vi "Stop Acquisition.vi"(8 "error in (no error)":errorcluster, 11 "Cluster":T1={"Camera.lvclass"=refnum, "InClusTiming 2"={"Pixelclock"=24, "Exposure"=46.39115, "ExposureTimeBase"=2, "Framerate"=14.99615, "TriggerMode"=0}, "ROI"={"PosX"=0, "PosY"=0, "Width"=0, "Height"=0}, "File Path Control"=path "", "mirror.lvclass"=refnum} {"InClusTiming 2"."TriggerMode" items=["Auto", "Software", "External sequence start ", "External exposure control"]; "InClusTiming 2"."ExposureTimeBase" items=["nanoseconds", "microseconds", "milliseconds"]; "InClusTiming 2"."Pixelclock" min=1 max=400 step=1 scale=0.05915..400.0 scale format="%#.3g"; "InClusTiming 2"."Framerate" min=0.05915 max=2000.0 step=1.0 scale=0.05915..100.0 scale format="%#.3g"; "InClusTiming 2"."Exposure" min=0.05915 max=2000.0 step=1.0 scale=0.05915..100.0 scale format="%#.3g"}) -> (0 "error out":errorcluster, 3 "Cluster":T1={"Camera.lvclass"=refnum, "InClusTiming 2"={"Pixelclock"=24, "Exposure"=46.39115, "ExposureTimeBase"=2, "Framerate"=14.99615, "TriggerMode"=0}, "ROI"={"PosX"=0, "PosY"=0, "Width"=0, "Height"=0}, "File Path Control"=path "", "mirror.lvclass"=refnum} {"InClusTiming 2"."TriggerMode" items=["Auto", "Software", "External sequence start ", "External exposure control"]; "InClusTiming 2"."ExposureTimeBase" items=["nanoseconds", "microseconds", "milliseconds"]; "InClusTiming 2"."Pixelclock" min=1 max=400 step=1 scale=0.05915..400.0 scale format="%#.3g"; "InClusTiming 2"."Framerate" min=0.05915 max=2000.0 step=1.0 scale=0.05915..100.0 scale format="%#.3g"; "InClusTiming 2"."Exposure" min=0.05915 max=2000.0 step=1.0 scale=0.05915..100.0 scale format="%#.3g"})   [LabVIEW 2020, in "Acquisition.lvlib"]
doc: "Stops the acquisition."
uses:
  Acquisition.lvlib
  HardwareConfiguration.ctl
  CLASS/Image Acquisition Class/Camera.lvclass
  MIRROR/mirror.lvclass
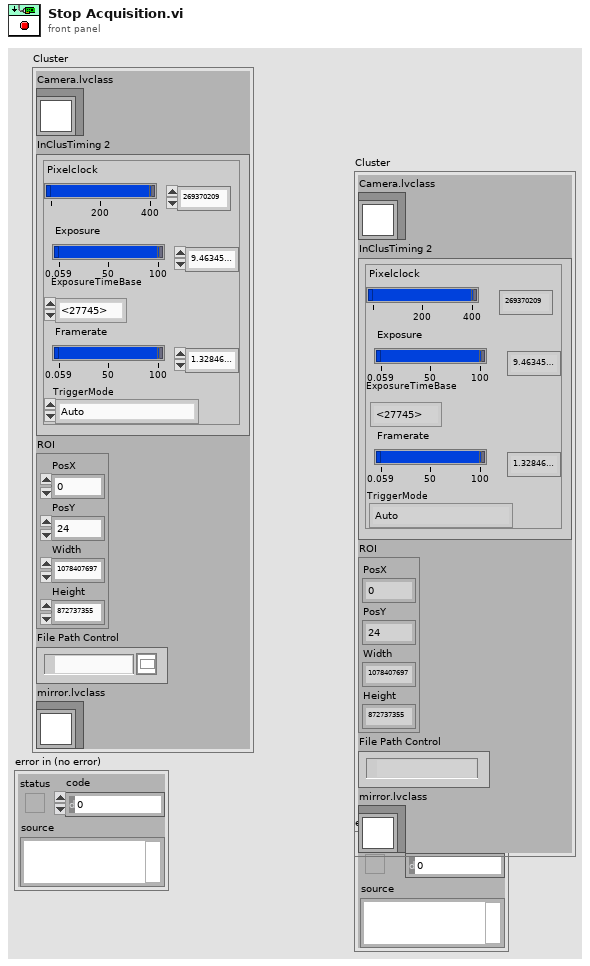
[diagram p1: front panel]
types:
  T1 = typedef "Acquisition.lvlib/HardwareConfiguration.ctl" = cluster{"Camera.lvclass":refnum<class "Camera.lvclass">, "InClusTiming 2":cluster{"Pixelclock":i32, "Exposure":dbl, "ExposureTimeBase":u16, "Framerate":dbl, "TriggerMode":u16}, "ROI":cluster{"PosX":i32, "PosY":i32, "Width":i32, "Height":i32}, "File Path Control":path, "mirror.lvclass":refnum<class "mirror.lvclass">}
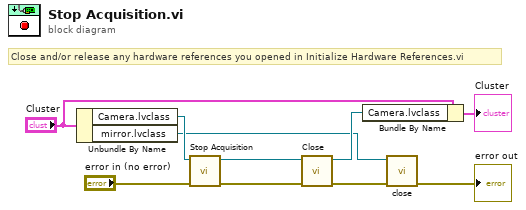
[diagram p0: block diagram]
diagram:
  # "Close and/or release any hardware references you opened in Initialize Hardware References.vi"
  n1 = Unbundle By Name("Cluster") -> ("Camera.lvclass"=w6:refnum<class "Camera.lvclass">, "mirror.lvclass"=w2:refnum<class "mirror.lvclass">)
  n2 = call-dynamic "Stop Acquisition.vi"("error in (no error)"="error in (no error)", "Camera in"=w6) -> ("error out"=w9:errorcluster, "Camera out"=w8:refnum<class "Camera.lvclass">)  [unwired: 8 in]
  n3 = call-dynamic "Close.vi"("error in (no error)"=w9, "Camera in"=w8) -> ("error out"=w3:errorcluster, "Camera out"=w4:refnum<class "Camera.lvclass">)  [unwired: 8 in]
  n4 = Bundle By Name(cluster="Cluster", "Camera.lvclass"=w4) -> (→"Cluster":T1)
  n5 = call-dynamic "close.vi"("error in (no error)"=w3, "mirror in"=w2) -> ("error out"=→"error out":errorcluster)  [unwired: 8 in, 1 out]
